vi "XY Graph Check New Plot Name.vi"(8 "Error In":errorcluster, 9 "New Plot Name (in)":string, 11 "Multiplot XY Graph Refnum in":T1) -> (0 "Error Out":errorcluster, 1 "New Plot Name (out)":string, 3 "Multiplot XY Graph Refnum out":T1)   [LabVIEW 2021, in "XY Graph Add-Ons.lvlib"]
uses:
  XY Graph Refnum.ctl
  XY Graph Add-Ons.lvlib
  Strings/Strings.lvlib
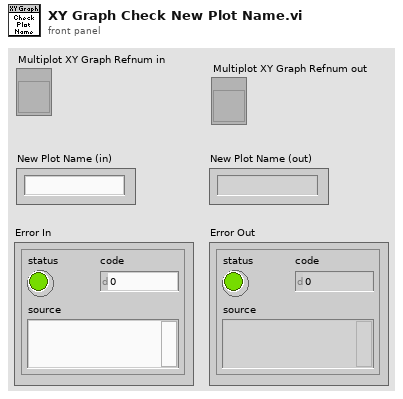
[diagram p1: front panel]
types:
  T1 = typedef "XY Graph Add-Ons.lvlib/XY Graph Refnum.ctl" = refnum<vi>
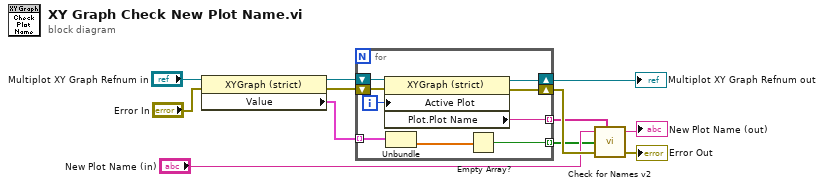
[diagram p0: block diagram]
diagram:
  n1 = property class="XYGraph (strict)"(reference="Multiplot XY Graph Refnum in", error in="Error In") -> (reference out=w11:T1, error out=w10:errorcluster, "Value"=w2:cluster{"X Array":dbl[], "Y Array":dbl[]}[])
  n2 = for {
    tunnel: [w19] -> w6 mode=indexing
    shift-right: [w17] -> w8
    shift-left: w10 -> [w18]
    shift-right: [w16] -> w7
    shift-left: w11 -> [w21]
    tunnel: w2 -> [w15] mode=indexing
    tunnel: [w13] -> w1 mode=indexing
    i -> [w20]
    n3 = property class="XYGraph (strict)"(reference=w21, error in=w18, "Active Plot"=w20) -> (reference out=w16:T1, error out=w17:errorcluster, "Plot.Plot Name"=w19:string)
    n4 = Unbundle(w15) -> ("Y Array"=w14:dbl[])  [unwired: 1 out]
    n5 = Empty Array?(array=w14) -> (empty?=w13:bool)
  }
  "Multiplot XY Graph Refnum out" <- w7
  n6 = call "Check for Names v2.vi"("New Name"="New Plot Name (in)", "Name List"=w6, "Empty Plots?"=w1, "Error In"=w8) -> ("New Name"=→"New Plot Name (out)":string, "Error Out"=→"Error Out":errorcluster)  [unwired: 2 in, 2 out]
